vi "Inv T Distribution.vi"(2 "degrees of freedom":i32=1, 3 "probability":dbl format="%0.4f") -> (0 "error":i32, 1 "x":dbl format="%0.4f")   [LabVIEW 2017, in "NI_AALPro.lvlib"]
doc: "LabVIEW no longer supports this VI. Use the Continuous Inverse CDF VI (T instance) instead. Computes the one-tailed t value of <B>x</B>. The Inv T Distribution VI computes the one-tailed t value of <B>x</B> such that the following condition is satisfied: p = Prob{T[n] <= <B>x</B>} given the <B>probability</B> value, (1 - p), of a t-distributed random variable, T, with n <B>degrees of freedom</B>."
uses:
  <vilib>/Analysis/NI_AALPro.lvlib
  <resource>/lvanlys.dll
panel:
  # "Inverse t Distribution"
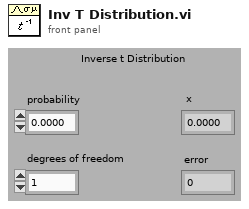
[diagram p1: front panel]
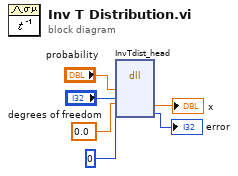
[diagram p0: block diagram]
diagram:
  n1 = dll-call lib="e:/builds/penguin/labview/branches/2017/dev/dist/resource/lvanlys.*" fn="InvTdist_head"("probability"="probability", "degrees of freedom"="degrees of freedom", 0.0, 0) -> (→"x":dbl, →"error":i32)  [unwired: 6 in, 2 out]
